vi "BRig_RT__Case_Exp__clearLocalFolder.vi"   [LabVIEW 2014]
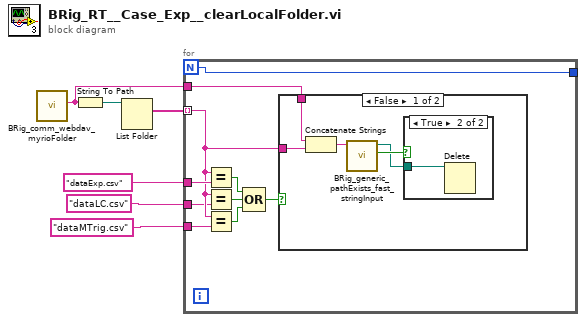
[diagram p0: block diagram]
diagram:
  n1 = call "BRig_comm_webdav_myrioFolder.vi"() -> ("output_myrioFolder"=w5:string)  [unwired: 11 in]
  n2 = String To Path(string=w5) -> (path=w4:path)
  n3 = List Folder(path=w4) -> (filenames=w6:string[])  [unwired: 3 in, 3 out]
  n4 = for {
    N -> [w15]
    tunnel: w6 -> [w13] mode=indexing
    tunnel: w5 -> [w16]
    tunnel: [w15] -> _
    tunnel: "dataExp.csv" ("y") -> [w14]
    tunnel: "dataLC.csv" ("y") -> [w12]
    tunnel: "dataMTrig.csv" ("y") -> [w11]
    n5 = Equal?(x=w13, y=w14) -> (x = y?=w9:bool)
    n6 = Equal?(x=w13, y=w12) -> (x = y?=w10:bool)
    n7 = Equal?(x=w13, y=w11) -> (x = y?=w8:bool)
    n8 = Compound Arithmetic op=OR(w9, w10, w8) -> (w7:bool)
    n9 = case shown="False" w7 {
      tunnel: w16 -> [w21 _]
      tunnel: w13 -> [w17 _]
      frame False {
        n10 = Concatenate Strings(w21, w17) -> (w20:string)
        n11 = call "BRig_generic_pathExists_fast_stringInput.vi"("input_filePath"=w20) -> ("output_Iexist"=w19:bool, "output_filePath"=w18:path)  [unwired: 8 in, 1 out]
        n12 = case shown="True" w19 {
          tunnel: w18 -> [_ w22]
          frame False {
          }
          frame True {
            n13 = Delete(path (use dialog)=w22) -> ()  [unwired: 4 in, 3 out]
          }
        }
      }
      frame True {
      }
    }
  }
